vi "Calibration_Save.vi"(0 "Img1":T4, 1 "Data":T1={"Pinch-valve"="", "XLP 6000 Pump"="", "Camera1"="", "Camera2"="", "Img_Capt"=FALSE, "Actuator"=FALSE, "Pump"=FALSE, "Cam 1"=FALSE, "Cam 2"=FALSE, "Empty_Refill"=FALSE, "Crop"=FALSE, "Light intensity"=0, "Exposure Time"=0.0, "Sample Name"="", "Operator"="", "Calibration 1"=path "", "Calibration 2"=path "", "Framerate"=0, "Timeout Sample"=1, "Collection date"="", "Sample size threshold"=500, "Empty start"=500, "Command"="", "Station"="", "Species Name"="", "Other Notes"="", "Aperture"=enum."Item 3", "Image Process Queue Size"=100, "Image Save Queue Size"=0, "Overload threshold"=0, "Max Framerate"=0, "Rectangle 1"={"Left"=0, "Top"=0, "Right"=0, "Bottom"=0, "Rotation"=0.0}, "Rectangle 2"={"Left"=0, "Top"=100, "Right"=100, "Bottom"=0, "Rotation"=0.0}, "Detection Region %"=200.0, "Detect 1"=path "C:/Users/au540322/Desktop/IHS_Project/images/Debris/Debris_0/Debris_0_2019_06_01-23-32-49-686.PNG", "Detect 2"=path "C:/Users/au540322/Desktop/IHS_Project/images/Debris/Debris_0/Debris_0_2019_06_01-23-32-49-686.PNG", "Max large object threshold"=500, "Open(T)/Close(F)"=FALSE, "Img_Capt Begin"=FALSE, "Dispense Speed"=0, "Flush Size"=0, "Location"="", "Latitude"="", "Longitude"="", "Determiner"="", "Sex"="", "Camera1_Img"=refnum, "Camera2_Img"=refnum, "Img1_Orig_Disp"=refnum, "Img2_Orig_Disp"=refnum, "Img1_Orig_RGB"=refnum, "Img2_Orig_RGB"=refnum, "Blue_Plane_Extract"=refnum, "Subtracted_Plane"=refnum, "Img1_Binary"=refnum, "Img2_Binary"=refnum, "Crop_Mask"=refnum, "Img1_Save"=refnum, "Img2_Save"=refnum, "Img1_Cali_Full"=refnum, "Img2_Cali_Full"=refnum, "Img1_Cali_Detect"=refnum, "Img2_Cali_Detect"=refnum, "Cam 1 queue"=refnum, "Cam 2 queue"=refnum, "Cam 1 - save queue"=refnum, "Cam 2 - save queue"=refnum, "Overlay_Ring"=0, "SystemVersion"=0, "System Serial"="", "Legacy Cam Attributes"=FALSE, "Camera Orientation 1"="", "Camera Orientation 2"="", "Pixel to mm 1"=0.0, "Pixel to mm 2"=0.0} {"SystemVersion" items=["Standard", "XL"]; "Overlay_Ring" items=["Session Data", "Extended Setup", "Buffer", "Camera", "Dispenser", "Stats", "Connections"]; "Flush Size" min=1; "Dispense Speed" min=1; "Rectangle 2"."Rotation" format="%.2f"; "Rectangle 2"."Left" scale=0.0..1024.0; "Rectangle 2"."Right" scale=0.0..1024.0; "Rectangle 1"."Rotation" format="%.2f"; "Rectangle 1"."Left" scale=0.0..1024.0; "Rectangle 1"."Right" scale=0.0..1024.0; "Max Framerate" min=1; "Overload threshold" min=1; "Image Save Queue Size" min=1; "Image Process Queue Size" min=1; "Empty start" min=1; "Sample size threshold" min=1; "Framerate" min=1; "Light intensity" scale=0.0..100.0}, 5 "Img2":T4, 9 "Dtct":bool, 11 "Crop?":bool) -> (4 "Cal1":path, 6 "Cal2":path, 8 "Data out":T1={"Pinch-valve"="", "XLP 6000 Pump"="", "Camera1"="", "Camera2"="", "Img_Capt"=FALSE, "Actuator"=FALSE, "Pump"=FALSE, "Cam 1"=FALSE, "Cam 2"=FALSE, "Empty_Refill"=FALSE, "Crop"=FALSE, "Light intensity"=0, "Exposure Time"=0.0, "Sample Name"="", "Operator"="", "Calibration 1"=path "", "Calibration 2"=path "", "Framerate"=0, "Timeout Sample"=1, "Collection date"="", "Sample size threshold"=500, "Empty start"=500, "Command"="", "Station"="", "Species Name"="", "Other Notes"="", "Aperture"=enum."Item 3", "Image Process Queue Size"=100, "Image Save Queue Size"=0, "Overload threshold"=0, "Max Framerate"=0, "Rectangle 1"={"Left"=0, "Top"=0, "Right"=0, "Bottom"=0, "Rotation"=0.0}, "Rectangle 2"={"Left"=0, "Top"=100, "Right"=100, "Bottom"=0, "Rotation"=0.0}, "Detection Region %"=200.0, "Detect 1"=path "C:/Users/au540322/Desktop/IHS_Project/images/Debris/Debris_0/Debris_0_2019_06_01-23-32-49-686.PNG", "Detect 2"=path "C:/Users/au540322/Desktop/IHS_Project/images/Debris/Debris_0/Debris_0_2019_06_01-23-32-49-686.PNG", "Max large object threshold"=500, "Open(T)/Close(F)"=FALSE, "Img_Capt Begin"=FALSE, "Dispense Speed"=0, "Flush Size"=0, "Location"="", "Latitude"="", "Longitude"="", "Determiner"="", "Sex"="", "Camera1_Img"=refnum, "Camera2_Img"=refnum, "Img1_Orig_Disp"=refnum, "Img2_Orig_Disp"=refnum, "Img1_Orig_RGB"=refnum, "Img2_Orig_RGB"=refnum, "Blue_Plane_Extract"=refnum, "Subtracted_Plane"=refnum, "Img1_Binary"=refnum, "Img2_Binary"=refnum, "Crop_Mask"=refnum, "Img1_Save"=refnum, "Img2_Save"=refnum, "Img1_Cali_Full"=refnum, "Img2_Cali_Full"=refnum, "Img1_Cali_Detect"=refnum, "Img2_Cali_Detect"=refnum, "Cam 1 queue"=refnum, "Cam 2 queue"=refnum, "Cam 1 - save queue"=refnum, "Cam 2 - save queue"=refnum, "Overlay_Ring"=0, "SystemVersion"=0, "System Serial"="", "Legacy Cam Attributes"=FALSE, "Camera Orientation 1"="", "Camera Orientation 2"="", "Pixel to mm 1"=0.0, "Pixel to mm 2"=0.0} {"SystemVersion" items=["Standard", "XL"]; "Overlay_Ring" items=["Session Data", "Extended Setup", "Buffer", "Camera", "Dispenser", "Stats", "Connections"]; "Flush Size" min=1; "Dispense Speed" min=1; "Rectangle 2"."Rotation" format="%.2f"; "Rectangle 2"."Left" scale=0.0..1024.0; "Rectangle 2"."Right" scale=0.0..1024.0; "Rectangle 1"."Rotation" format="%.2f"; "Rectangle 1"."Left" scale=0.0..1024.0; "Rectangle 1"."Right" scale=0.0..1024.0; "Max Framerate" min=1; "Overload threshold" min=1; "Image Save Queue Size" min=1; "Image Process Queue Size" min=1; "Empty start" min=1; "Sample size threshold" min=1; "Framerate" min=1; "Light intensity" scale=0.0..100.0}, 10 "Img1 out":T4, 15 "Img2 out":T4)   [LabVIEW 2022 SP3]
uses:
  controls/Data.ctl
  <vilib>/userdefined/High Color/IMAQdx.ctl
  <vilib>/vision/Image Controls.llb/IMAQ Image.ctl
panel:
  out "error out 2":errorcluster
  out "error out":errorcluster
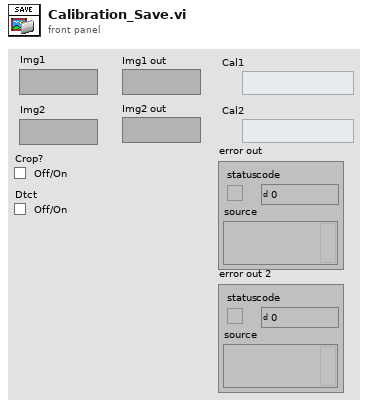
[diagram p1: front panel]
types:
  T1 = typedef "Data.ctl" = cluster{"Pinch-valve":refnum<visa-resource-name>, "XLP 6000 Pump":refnum<visa-resource-name>, "Camera1":T2, "Camera2":T2, "Img_Capt":bool, "Actuator":bool, "Pump":bool, "Cam 1":bool, "Cam 2":bool, "Empty_Refill":bool, "Crop":bool, "Light intensity":i32, "Exposure Time":dbl, "Sample Name":string, "Operator":string, "Calibration 1":path, "Calibration 2":path, "Framerate":i32, "Timeout Sample":i32, "Collection date":string, "Sample size threshold":i32, "Empty start":u32, "Command":string, "Station":string, "Species Name":string, "Other Notes":string, "Aperture":enum32{"Item 0", "Item 1", "Item 2", "Item 3"}, "Image Process Queue Size":i32, "Image Save Queue Size":i32, "Overload threshold":i32, "Max Framerate":i32, "Rectangle 1":T3, "Rectangle 2":T3, "Detection Region %":dbl, "Detect 1":path, "Detect 2":path, "Max large object threshold":i32, "Open(T)/Close(F)":bool, "Img_Capt Begin":bool, "Dispense Speed":i32, "Flush Size":i32, "Location":string, "Latitude":string, "Longitude":string, "Determiner":string, "Sex":string, "Camera1_Img":T4, "Camera2_Img":T4, "Img1_Orig_Disp":T4, "Img2_Orig_Disp":T4, "Img1_Orig_RGB":T4, "Img2_Orig_RGB":T4, "Blue_Plane_Extract":T4, "Subtracted_Plane":T4, "Img1_Binary":T4, "Img2_Binary":T4, "Crop_Mask":T4, "Img1_Save":T4, "Img2_Save":T4, "Img1_Cali_Full":T4, "Img2_Cali_Full":T4, "Img1_Cali_Detect":T4, "Img2_Cali_Detect":T4, "Cam 1 queue":refnum<queue>, "Cam 2 queue":refnum<queue>, "Cam 1 - save queue":refnum<queue>, "Cam 2 - save queue":refnum<queue>, "Overlay_Ring":u16, "SystemVersion":u16, "System Serial":string, "Legacy Cam Attributes":bool, "Camera Orientation 1":string, "Camera Orientation 2":string, "Pixel to mm 1":dbl, "Pixel to mm 2":dbl}
  T2 = typedef "IMAQdx.ctl" = refnum<k21>
  T3 = typedef "IMAQ Rectangle" = cluster{"Left":i32, "Top":i32, "Right":i32, "Bottom":i32, "Rotation":dbl}
  T4 = typedef "IMAQ Image.ctl" = refnum<image>
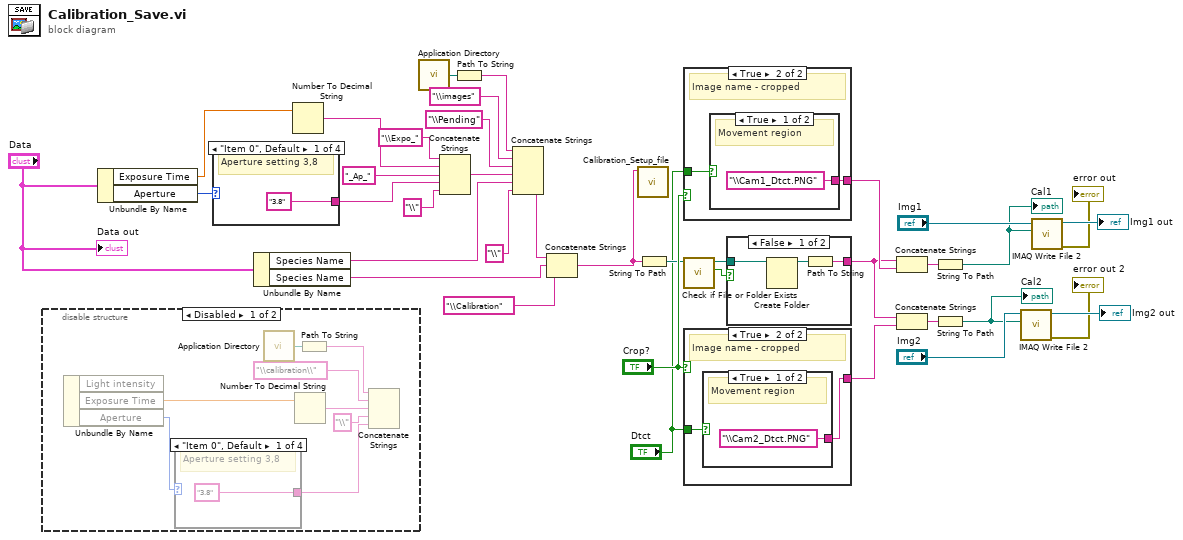
[diagram p0: block diagram]
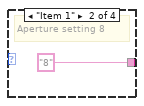
[diagram p2: hidden frame]
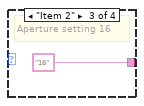
[diagram p3: hidden frame]
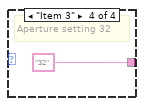
[diagram p4: hidden frame]
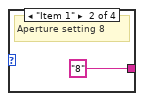
[diagram p6: hidden frame]
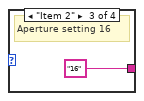
[diagram p7: hidden frame]
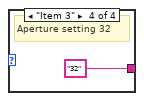
[diagram p8: hidden frame]
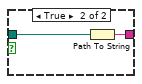
[diagram p9: hidden frame]
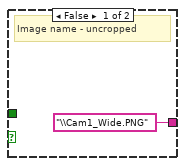
[diagram p10: hidden frame]
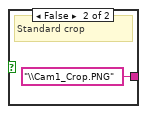
[diagram p11: hidden frame]
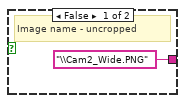
[diagram p12: hidden frame]
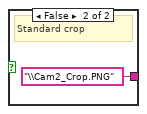
[diagram p13: hidden frame]
diagram:
  n1 = disable-structure shown="Disabled" {
    frame Disabled {
      n2 = Unbundle By Name() -> ("Exposure Time"=w44:dbl, "Aperture"=w38:enum32{"Item 0", "Item 1", "Item 2", "Item 3"})  [unwired: 1 in, 1 out]
      n3 = case shown="\"Item 0\", Default" w38 {
        tunnel: ["3.8" "8" "16" "32"] -> w39
        frame "Item 0", Default {
          # "Aperture setting 3,8"
        }
        frame "Item 1" {
          # "Aperture setting 8"
        }
        frame "Item 2" {
          # "Aperture setting 16"
        }
        frame "Item 3" {
          # "Aperture setting 32"
        }
      }
      n4 = call <vilib>:"Application Directory.vi"() -> ("Application Directory"=w41:path)
      n5 = Number To Decimal String(number=w44) -> (decimal integer string=w43:string)  [unwired: 1 in]
      n6 = Path To String(path=w41) -> (string=w40:string)
      n7 = Concatenate Strings(w40, "\\calibration\\" ("string"), w43, "\\" ("string"), w39) -> ()  [unwired: 1 out]
    }
    frame Enabled {
    }
  }
  n8 = Unbundle By Name("Data") -> ("Exposure Time"=w24:dbl, "Aperture"=w21:enum32{"Item 0", "Item 1", "Item 2", "Item 3"})
  n9 = case shown="\"Item 0\", Default" w21 {
    tunnel: ["3.8" "8" "16" "32"] -> w19
    frame "Item 0", Default {
      # "Aperture setting 3,8"
    }
    frame "Item 1" {
      # "Aperture setting 8"
    }
    frame "Item 2" {
      # "Aperture setting 16"
    }
    frame "Item 3" {
      # "Aperture setting 32"
    }
  }
  n10 = Unbundle By Name("Data") -> ("Species Name"=w28:string, "Species Name"=w26:string)
  n11 = Number To Decimal String(number=w24) -> (decimal integer string=w20:string)  [unwired: 1 in]
  n12 = call <vilib>:"Application Directory.vi"() -> ("Application Directory"=w29:path)
  n13 = Concatenate Strings("\\Expo_" ("string"), w20, "_Ap_" ("string"), w19, "\\" ("string")) -> (w17:string)
  n14 = Path To String(path=w29) -> (string=w3:string)
  n15 = Concatenate Strings(w3, "\\images" ("string"), "\\Pending" ("string"), w17, w28, "\\" ("string")) -> (w27:string)
  n16 = Concatenate Strings(w27, w26, "\\Calibration" ("string")) -> (w16:string)
  n17 = call "Calibration_Setup_file.vi"("Path"=w16) -> ()  [unwired: 11 in]
  n18 = String To Path(string=w16) -> (path=w32:path)
  n19 = case shown="True" "Crop?" {
    tunnel: ["\\Cam1_Wide.PNG" ("string") w56] -> w36
    tunnel: "Dtct" -> [_ w55]
    frame False {
      # "Image name - uncropped"
    }
    frame True {
      # "Image name - cropped"
      n20 = case shown="True" w55 {
        tunnel: ["\\Cam1_Dtct.PNG" ("string") "\\Cam1_Crop.PNG" ("string")] -> w56
        frame True {
          # "Movement region"
        }
        frame False {
          # "Standard crop"
        }
      }
    }
  }
  n21 = call <vilib>:"Check if File or Folder Exists.vi"("path"=w32) -> ("file or folder exists?"=w34:bool, "dup path"=w33:path)  [unwired: 8 in, 1 out]
  n22 = case shown="True" "Crop?" {
    tunnel: ["\\Cam2_Wide.PNG" ("string") w61] -> w37
    tunnel: "Dtct" -> [_ w60]
    frame False {
      # "Image name - uncropped"
    }
    frame True {
      # "Image name - cropped"
      n23 = case shown="True" w60 {
        tunnel: ["\\Cam2_Dtct.PNG" ("string") "\\Cam2_Crop.PNG" ("string")] -> w61
        frame True {
          # "Movement region"
        }
        frame False {
          # "Standard crop"
        }
      }
    }
  }
  n24 = case shown="False" w34 {
    tunnel: w33 -> [w66 w68]
    tunnel: [w64 w67] -> w31
    frame False {
      n25 = Create Folder(path (use dialog)=w66) -> (created path=w65:path)  [unwired: 2 in, 2 out]
      n26 = Path To String(path=w65) -> (string=w64:string)
    }
    frame True {
      n27 = Path To String(path=w68) -> (string=w67:string)
    }
  }
  n28 = Concatenate Strings(w31, w36) -> (w12:string)
  n29 = Concatenate Strings(w31, w37) -> (w13:string)
  n30 = String To Path(string=w12) -> (path=w9:path)
  "Cal1" <- w9
  n31 = String To Path(string=w13) -> (path=w8:path)
  "Cal2" <- w8
  n32 = call-poly "IMAQ Write File 2"("File Path"=w8, "Image"="Img2") -> ("error out"=→"error out 2":errorcluster, "Image Out (duplicate)"=→"Img2 out":T4)  [unwired: 8 in]
  n33 = call-poly "IMAQ Write File 2"("File Path"=w9, "Image"="Img1") -> ("error out"=→"error out":errorcluster, "Image Out (duplicate)"=→"Img1 out":T4)  [unwired: 8 in]
  "Data out" <- "Data"
